vi "asset.from_json.vi"(8 "error in":errorcluster, 10 "asset":string) -> (0 "error out":errorcluster, 2 "Asset Data":T7)   [LabVIEW 2020, in "asset.lvclass"]
uses:
  asset.lvclass
  nominal types/properties/properties.lvclass
  nominal types/labels/labels.lvclass
  nominal types/dataScope/links.ctl
  nominal types/dataScope/data_scopes.ctl
  nominal types/dataScope/data_scope.ctl
  nominal types/dataScope/data_source.ctl
  nominal types/dataScope/type.ctl
  nominal types/dataScope/offset.ctl
  asset.lvclass/asset.ctl
  02f22241-51c4-4473-a36f-78f3127849f2.vi
  bfdfcee5-81ab-4956-b6ce-ad5bee6cacef.vi
  856e22dd-e93b-4c21-b825-9b1f5d095f0e.vi
  582e419f-de3c-4dbc-8ecf-df929f928f55.vi
  97b0fc54-f6bc-4c4f-b7ab-356d389efbe9.vi
  73a2c702-0eb7-401a-afb6-8e357fc678eb.vi
  362a07b5-d5ef-4f04-8007-9594c2c726f8.vi
  18bbe2ca-1498-4f7a-80b6-98471bfcd25a.vi
  9ada0a1a-2184-4ddd-b537-4dbb756a36f8.vi
  <vilib>/JDP Science/JSONtext/Find Item.vi
  <vilib>/JDP Science/JSONtext/String Subset.vi
  <vilib>/JDP Science/JSONtext/Offset/Find Object Item Locations by Names.vi
  <vilib>/JDP Science/JSONtext/support/Quote and Escape JSON string.vi
  <vilib>/JDP Science/JSONtext/Next JSON Value.vi
  <vilib>/JDP Science/JSONtext/Parsing/Advance past whitespace.vi
  <vilib>/JDP Science/JSONtext/support/Commas Needed.vi
  <vilib>/JDP Science/JSONtext/Parsing/Advance past whitespace and comma.vi
  <vilib>/JDP Science/JSONtext/Parsing/Advance past next JSON Value (inlined COPY).vi
  <vilib>/JDP Science/JSONtext/Parsing/Advance past Item Name.vi
  <vilib>/JDP Science/JSONtext/support/quote and escape json string 2.vi
  <vilib>/JDP Science/JSONtext/Parsing/Advance past Line Ending.vi
  <vilib>/JDP Science/JSONtext/Parsing/Advance past String.vi
  <vilib>/JDP Science/JSONtext/Parsing/Advance past Number.vi
  <vilib>/JDP Science/JSONtext/Parsing/Parse Full Path or Item Name.vi
  <vilib>/JDP Science/JSONtext/Parsing/Advance past Array.vi
  <vilib>/JDP Science/JSONtext/Parsing/Advance past Object.vi
  <vilib>/JDP Science/JSONtext/support/Error Cluster From Code.vi
  <vilib>/JDP Science/JSONtext/Offset/Find Item Locations by Path.vi
  <vilib>/JDP Science/JSONtext/Parsing/Parsing Error.vi
  <vilib>/JDP Science/JSONtext/JSON text to Variant.vi
  <vilib>/LabVIEW Open Source Project/Epoch Date & Time/formatter.iso8601/ISO8601 DateString to Timestamp.vi
  <vilib>/JDP Science/JSONtext/LVClass Serializer/JSONtext LVClass Serializer.lvclass
  <vilib>/JDP Science/JSONtext/JSONtext.lvlib
  Nominal Client/Nominal Client.lvclass
  nominal types/dataScope/dataScopes.lvlib
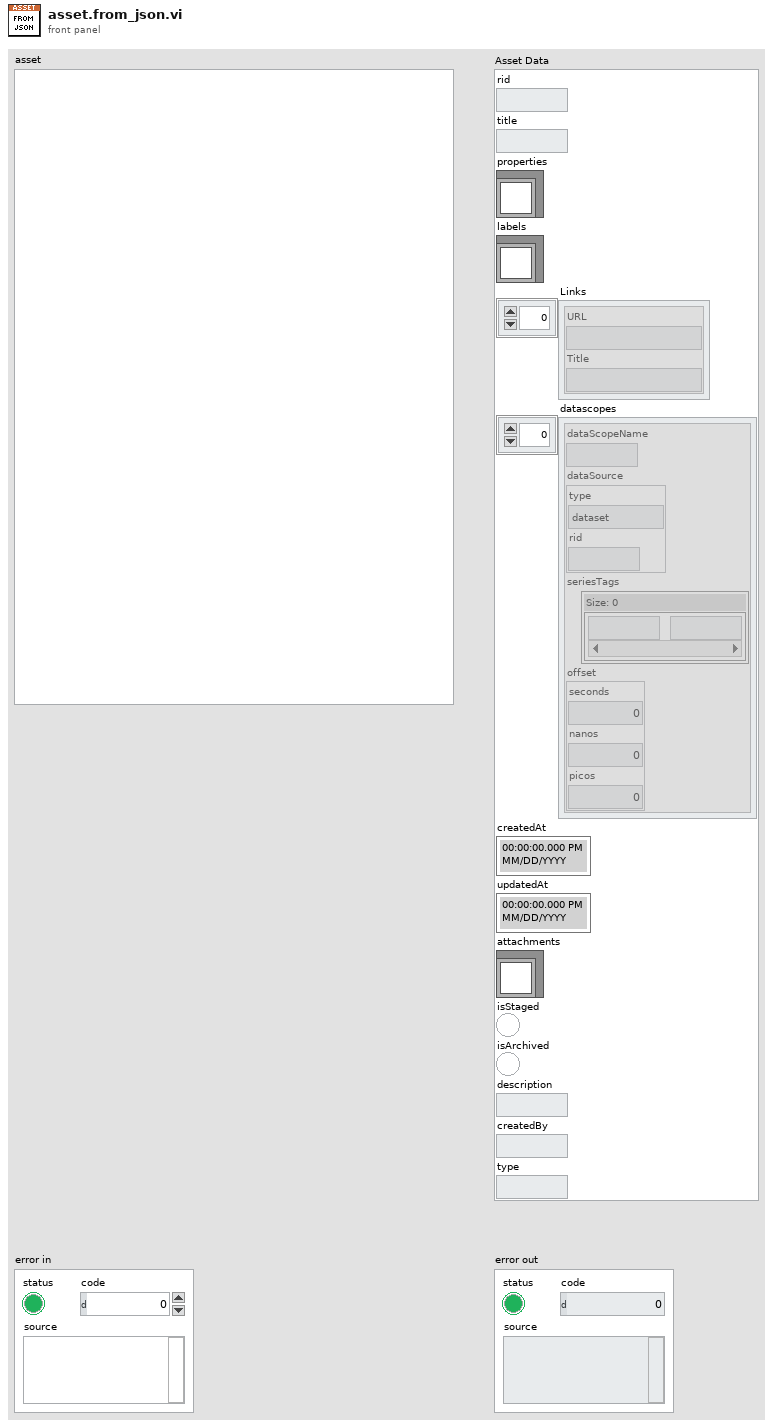
[diagram p1: front panel]
types:
  T1 = typedef "dataScopes.lvlib/links.ctl" = cluster{"URL":string, "Title":string}[]
  T2 = typedef "dataScopes.lvlib/data_scopes.ctl" = T3[]
  T3 = typedef "dataScopes.lvlib/data_scope.ctl" = cluster{"dataScopeName":string, "dataSource":T4, "seriesTags":map{string, string}, "offset":T6}
  T4 = typedef "dataScopes.lvlib/data_source.ctl" = cluster{"type":T5, "rid":string}
  T5 = typedef "dataScopes.lvlib/type.ctl" = enum16{"dataset", "connection", "logSet", "video"}
  T6 = typedef "dataScopes.lvlib/offset.ctl" = cluster{"seconds":i32, "nanos":i32, "picos":i32}
  T7 = cluster{"rid":string, "title":string, "properties":refnum<class "properties.lvclass">, "labels":refnum<class "labels.lvclass">, "Links":T1, "datascopes":T2, "createdAt":timestamp, "updatedAt":timestamp, "attachments":refnum<class "labels.lvclass">, "isStaged":bool, "isArchived":bool, "description":string, "createdBy":string, "type":string}
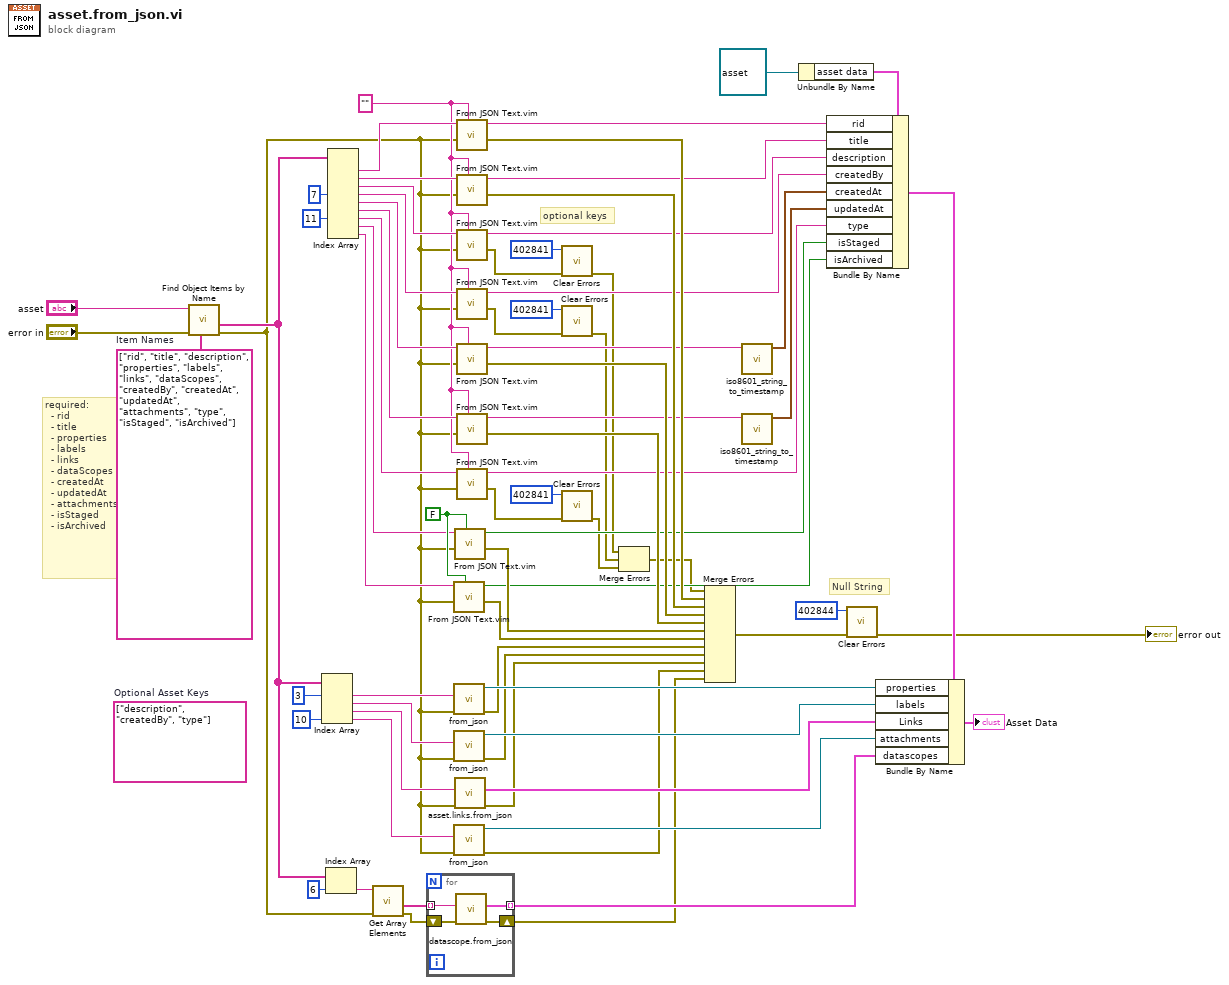
[diagram p0: block diagram]
diagram:
  w11 = string[] ["rid", "title", "description", "properties", "labels", "links", "dataScopes", "createdBy", "createdAt", "updatedAt", "attachments", "type", "isStaged", "isArchived"]  # Item Names
  (unwired) string[] ["description", "createdBy", "type"]  # Optional Asset Keys
  w45 = FALSE
  w52 = "" ("JSON")
  # "optional keys"
  # "required:\n  - rid\n  - title\n  - properties\n  - labels\n  - links\n  - dataScopes\n  - createdAt\n  - updatedAt\n  - attachments\n  - isStaged\n  - isArchived"
  # "Null String"
  n1 = call <vilib>:"Find Object Items by Name.vi"("Item Names"=w11, "error in (no error)"="error in", "JSON"="asset") -> ("error out"=w22:errorcluster, "<JSON>"=w29:string[])  [unwired: 6 in, 1 out]
  n2 = Index Array(array=w29, index #1=3 ("index"), index #4=10 ("index")) -> (element #1=w39:string, element #2=w37:string, element #3=w35:string, element #4=w32:string)  [unwired: 2 in]
  n3 = Index Array(array=w29, index=6) -> (element=w26:string)
  n4 = Index Array(array=w29, index #4=7 ("index"), index #7=11 ("index")) -> (element #1=w64:string, element #2=w62:string, element #3=w63:string, element #4=w56:string, element #5=w55:string, element #6=w54:string, element #7=w53:string, element #8=w44:string, element #9=w43:string)  [unwired: 7 in]
  n5 = call <vilib>:"Get Array Elements.vi"("error in (no error)"=w22, "JSON"=w26) -> ("error out"=w23:errorcluster, "<JSON>"=w27:string[])  [unwired: 7 in, 1 out]
  n6 = for {
    tunnel: w27 -> [w76] mode=indexing
    tunnel: [w75] -> w25 mode=indexing
    shift-right: [w73] -> w17
    shift-left: w23 -> [w74]
    n7 = call "datascope.from_json.vi"("error in"=w74, "json"=w76) -> ("error out"=w73:errorcluster, "data scope"=w75:T3)  [unwired: 8 in]
  }
  n8 = call "From JSON Text.vim"("Data Type and Default Value"=w45, "error in (no error)"=w22, "JSON"=w43) -> ("error out"=w67:errorcluster, "Data out"=w42:bool)  [unwired: 7 in]
  n9 = call "from_json.vi"("error in"=w22, "json"=w39) -> ("error out"=w21:errorcluster, "properties out"=w38:refnum<class "properties.lvclass">)  [unwired: 8 in]
  n10 = call "from_json.vi"("error in"=w22, "json"=w37) -> ("error out"=w20:errorcluster, "labels out"=w36:refnum<class "labels.lvclass">)  [unwired: 8 in]
  n11 = call "from_json.vi"("error in"=w22, "json"=w32) -> ("error out"=w18:errorcluster, "labels out"=w31:refnum<class "labels.lvclass">)  [unwired: 8 in]
  n12 = call "From JSON Text.vim"("Data Type and Default Value"=w45, "error in (no error)"=w22, "JSON"=w44) -> ("error out"=w68:errorcluster, "Data out"=w41:bool)  [unwired: 7 in]
  n13 = call "asset.links.from_json.vi"("error in"=w22, "json"=w35) -> ("error out"=w19:errorcluster, "Links"=w34:T1)  [unwired: 8 in]
  n14 = call "From JSON Text.vim"("Data Type and Default Value"=w52, "error in (no error)"=w22, "JSON"=w64) -> ("error out"=w72:errorcluster, "Data out"=w61:string)  [unwired: 7 in]
  n15 = call "From JSON Text.vim"("Data Type and Default Value"=w52, "error in (no error)"=w22, "JSON"=w62) -> ("error out"=w71:errorcluster, "Data out"=w60:string)  [unwired: 7 in]
  n16 = call "From JSON Text.vim"("Data Type and Default Value"=w52, "error in (no error)"=w22, "JSON"=w63) -> ("error out"=w9:errorcluster, "Data out"=w59:string)  [unwired: 7 in]
  n17 = call "From JSON Text.vim"("Data Type and Default Value"=w52, "error in (no error)"=w22, "JSON"=w56) -> ("error out"=w5:errorcluster, "Data out"=w51:string)  [unwired: 7 in]
  n18 = call "From JSON Text.vim"("Data Type and Default Value"=w52, "error in (no error)"=w22, "JSON"=w55) -> ("error out"=w70:errorcluster, "Data out"=w50:string)  [unwired: 7 in]
  n19 = call "From JSON Text.vim"("Data Type and Default Value"=w52, "error in (no error)"=w22, "JSON"=w54) -> ("error out"=w69:errorcluster, "Data out"=w49:string)  [unwired: 7 in]
  n20 = call "From JSON Text.vim"("Data Type and Default Value"=w52, "error in (no error)"=w22, "JSON"=w53) -> ("error out"=w7:errorcluster, "Data out"=w46:string)  [unwired: 7 in]
  n21 = call <vilib>:"Clear Errors.vi"("error in (no error)"=w9, "specific error code to clear (0: all)"=402841) -> ("error out"=w4:errorcluster)  [unwired: 4 in, 1 out]
  n22 = call <vilib>:"Clear Errors.vi"("error in (no error)"=w5, "specific error code to clear (0: all)"=402841) -> ("error out"=w3:errorcluster)  [unwired: 4 in, 1 out]
  n23 = call <vilib>:"Clear Errors.vi"("error in (no error)"=w7, "specific error code to clear (0: all)"=402841) -> ("error out"=w2:errorcluster)  [unwired: 4 in, 1 out]
  n24 = Merge Errors(w4, w3, w2) -> (w1:errorcluster)
  n25 = Merge Errors(w1, w72, w71, w70, w69, w68, w67, w21, w20, w19, w18, w17) -> (w13:errorcluster)
  n26 = call "iso8601_string_to_timestamp.vi"("ISO8601 Timestamp String"=w50) -> ("Time Stamp"=w48:timestamp)  [unwired: 9 in, 1 out]
  n27 = call "iso8601_string_to_timestamp.vi"("ISO8601 Timestamp String"=w49) -> ("Time Stamp"=w47:timestamp)  [unwired: 9 in, 1 out]
  n28 = Unbundle By Name(refnum<class "asset.lvclass"> refnum ("asset")) -> ("asset data"=w24:T7)
  n29 = Bundle By Name(cluster=w24, "rid"=w61, "title"=w60, "description"=w59, "createdBy"=w51, "createdAt"=w48, "updatedAt"=w47, "type"=w46, "isStaged"=w41, "isArchived"=w42) -> (w30:T7)
  n30 = call <vilib>:"Clear Errors.vi"("error in (no error)"=w13, "specific error code to clear (0: all)"=402844) -> ("error out"=→"error out":errorcluster)  [unwired: 4 in, 1 out]
  n31 = Bundle By Name(cluster=w30, "properties"=w38, "labels"=w36, "Links"=w34, "attachments"=w31, "datascopes"=w25) -> (→"Asset Data":T7)
